vi "Error Code.vi"() -> (4 "Error Map":map{i32, string}(c390))   [LabVIEW 2024]
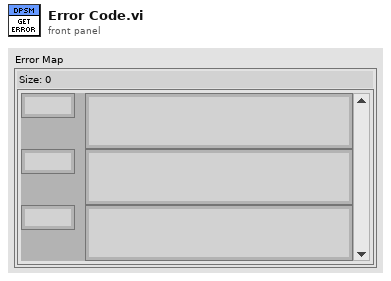
[diagram p1: front panel]
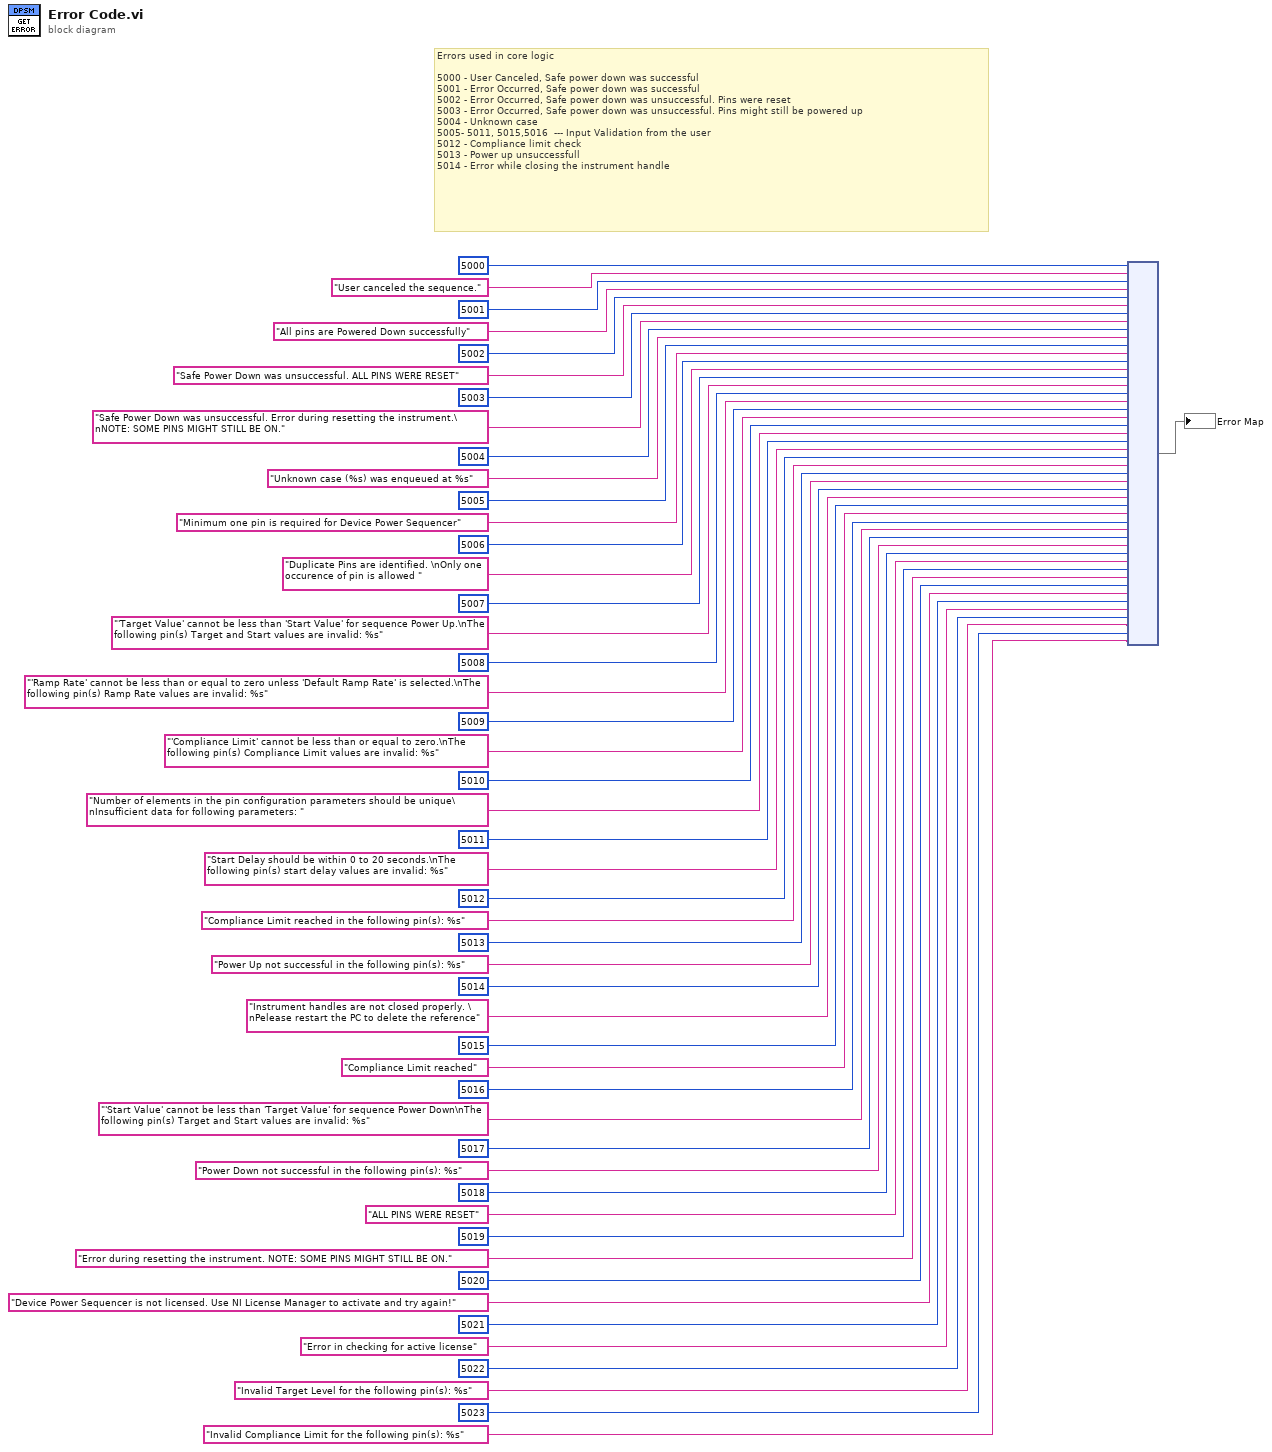
[diagram p0: block diagram]
diagram:
  # "Errors used in core logic\n\n5000 - User Canceled, Safe power down was successful\n5001 - Error Occurred, Safe power down was successful\n5002 - Error Occurred, Safe power down was unsuccessful. Pins were reset\n5003 - Error Occurred, Safe power down was unsuccessful. Pins might still be powered up\n5004 - Unknown case\n5005- 5011, 5015,5016  --- Input Validation from the user\n5012 - Compliance limit check\n5013 - Power up unsuccessfull\n5014 - Error while closing the instrument handle"
  n1 = node(5000 ("Error Code"), "User canceled the sequence.", 5001 ("Error Code"), "All pins are Powered Down successfully", 5002 ("Error Code"), "Safe Power Down was unsuccessful. ALL PINS WERE RESET", 5003 ("Error Code"), "Safe Power Down was unsuccessful. Error during resetting the instrument.\nNOTE: SOME PINS MIGHT STILL BE ON.", 5004 ("Error Code"), "Unknown case (%s) was enqueued at %s", 5005 ("Error Code"), "Minimum one pin is required for Device Power Sequencer" ("error message (\"\")"), 5006 ("error code (0)"), "Duplicate Pins are identified. \nOnly one occurence of pin is allowed " ("error message (\"\")"), 5007 ("error code (0)"), "'Target Value' cannot be less than 'Start Value' for sequence Power Up.\nThe following pin(s) Target and Start values are invalid: %s" ("error message (\"\")"), 5008 ("error code (0)"), "'Ramp Rate' cannot be less than or equal to zero unless 'Default Ramp Rate' is selected.\nThe following pin(s) Ramp Rate values are invalid: %s" ("error message (\"\")"), 5009 ("error code (0)"), "'Compliance Limit' cannot be less than or equal to zero.\nThe following pin(s) Compliance Limit values are invalid: %s" ("error message (\"\")"), 5010 ("error code (0)"), "Number of elements in the pin configuration parameters should be unique\nInsufficient data for following parameters: " ("error message (\"\")"), 5011 ("error code (0)"), "Start Delay should be within 0 to 20 seconds.\nThe following pin(s) start delay values are invalid: %s" ("error message (\"\")"), 5012 ("error code (0)"), "Compliance Limit reached in the following pin(s): %s" ("error message (\"\")"), 5013 ("error code (0)"), "Power Up not successful in the following pin(s): %s" ("error message (\"\")"), 5014 ("error code (0)"), "Instrument handles are not closed properly. \nPelease restart the PC to delete the reference" ("error message (\"\")"), 5015 ("error code (0)"), "Compliance Limit reached" ("error message (\"\")"), 5016 ("error code (0)"), "'Start Value' cannot be less than 'Target Value' for sequence Power Down\nThe following pin(s) Target and Start values are invalid: %s" ("error message (\"\")"), 5017 ("error code (0)"), "Power Down not successful in the following pin(s): %s" ("error message (\"\")"), 5018 ("error code (0)"), "ALL PINS WERE RESET" ("error message (\"\")"), 5019 ("error code (0)"), "Error during resetting the instrument. NOTE: SOME PINS MIGHT STILL BE ON." ("error message (\"\")"), 5020 ("error code (0)"), "Device Power Sequencer is not licensed. Use NI License Manager to activate and try again!" ("error message (\"\")"), 5021 ("error code (0)"), "Error in checking for active license" ("error message (\"\")"), 5022 ("error code (0)"), "Invalid Target Level for the following pin(s): %s" ("error message (\"\")"), 5023 ("error code (0)"), "Invalid Compliance Limit for the following pin(s): %s" ("error message (\"\")")) -> (→"Error Map":map{i32, string})
